vi "Cluster Autosize.vi"(8 "error in (no error)":errorcluster, 10 "AutoSize":T1(ring), 11 "GObject in":refnum<vi>) -> (0 "error out":errorcluster, 2 "is cluster?":bool, 3 "GObject out":refnum<vi>)   [LabVIEW 2019, in "Builtins.lvlib"]
doc: "Autosizes the selected cluster vertically, horizontally, size to fit or none.\n\nCreated by: Ryan Pacini"
uses:
  Builtins.lvlib
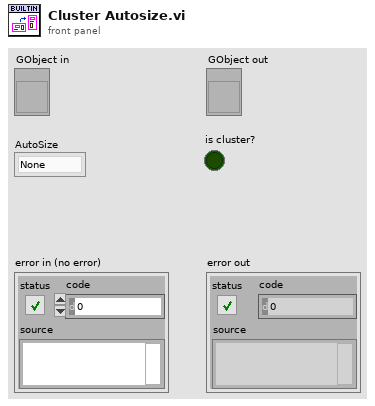
[diagram p1: front panel]
types:
  T1 = enum8{"None", "SizeToFit", "Horizontally", "Vertically"}
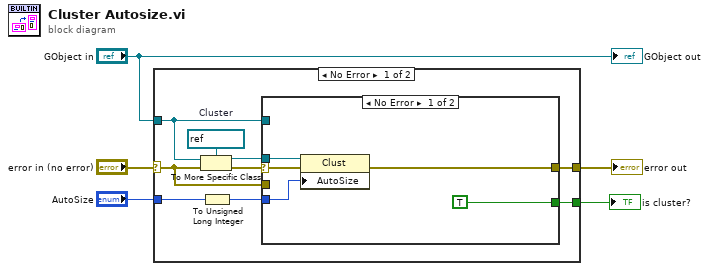
[diagram p0: block diagram]
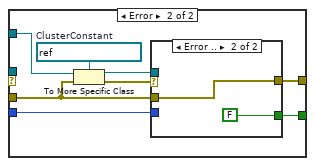
[diagram p2: hidden frame]
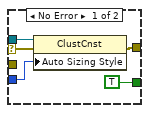
[diagram p3: hidden frame]
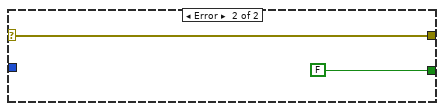
[diagram p4: hidden frame]
diagram:
  n1 = case shown="No Error" "error in (no error)" {
    selector: "error in (no error)" -> [w11 w36]
    tunnel: "GObject in" -> [w8 _]
    tunnel: [w10 w36] -> w4
    tunnel: "AutoSize" -> [w14 _]
    tunnel: [w6 FALSE] -> w1
    frame No Error {
      w12 = refnum<vi> refnum  # Cluster
      n2 = To More Specific Class(target class=w12, reference=w8, error in=w11) -> (specific class reference=w7:refnum<vi>, error out=w9:errorcluster)
      n3 = To Unsigned Long Integer(number=w14) -> (unsigned 32bit integer=w13:u32)
      n4 = case shown="No Error" w9 {
        selector: w9 -> [w19 _]
        tunnel: w13 -> [w17 w27]
        tunnel: w11 -> [_ w23]
        tunnel: [w16 w22] -> w10
        tunnel: w8 -> [_ w21]
        tunnel: w7 -> [w18 _]
        tunnel: [TRUE w20] -> w6
        frame No Error {
          n5 = property class="Clust"(reference=w18, error in=w19, "AutoSize"=w17) -> (error out=w16:errorcluster)  [unwired: 1 out]
        }
        frame Error {
          w25 = refnum<vi> refnum  # ClusterConstant
          n6 = To More Specific Class(target class=w25, reference=w21, error in=w23) -> (specific class reference=w26:refnum<vi>, error out=w24:errorcluster)
          n7 = case shown="Error .." w24 {
            selector: w24 -> [w31 _]
            tunnel: w26 -> [w32 _]
            tunnel: w27 -> [w30 _]
            tunnel: w23 -> [_ w34]
            tunnel: [w29 w34] -> w22
            tunnel: [TRUE FALSE] -> w20
            frame No Error {
              n8 = property class="ClustCnst"(reference=w32, error in=w31, "Auto Sizing Style"=w30) -> (error out=w29:errorcluster)  [unwired: 1 out]
            }
            frame Error {
            }
          }
        }
      }
    }
    frame Error {
    }
  }
  "error out" <- w4
  "is cluster?" <- w1
  "GObject out" <- "GObject in"
